vi "Param1.vi"(0 "str":refnum<vi>, 2 "Init_F":bool=TRUE, 5 "error in":errorcluster) -> (14 "str out":refnum<vi>, 19 "error out":errorcluster)   [LabVIEW 2010]
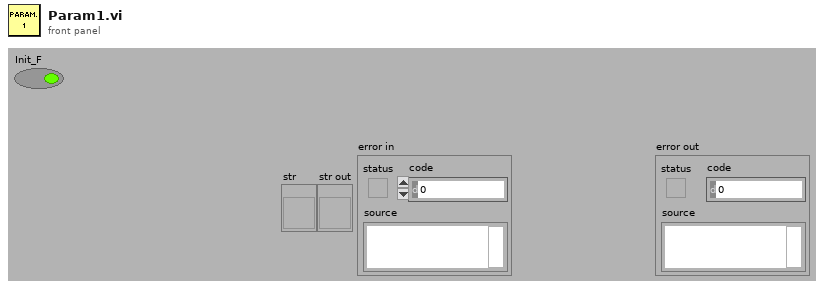
[diagram p1: front panel]
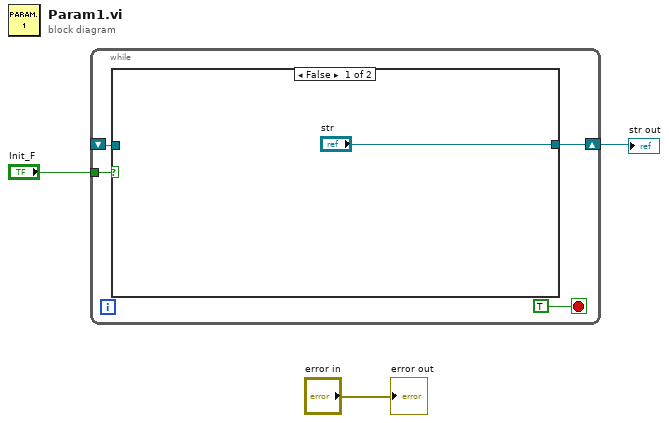
[diagram p0: block diagram]
diagram:
  n1 = while {
    shift-right: [w6] -> w2
    shift-left: _ -> [w5]
    tunnel: "Init_F" -> [w4]
    stop <- TRUE stop-if-true
    n2 = case shown="False" w4 {
      tunnel: ["str" w9] -> w6
      tunnel: w5 -> [_ w9]
      frame False {
      }
      frame True {
      }
    }
  }
  "str out" <- w2
  "error out" <- "error in"
